vi "能谱拼接.vi"(1 "数组":string[](array[string])) -> (0 "拼接数组":i32[](array[numeric]))   [LabVIEW 2014]
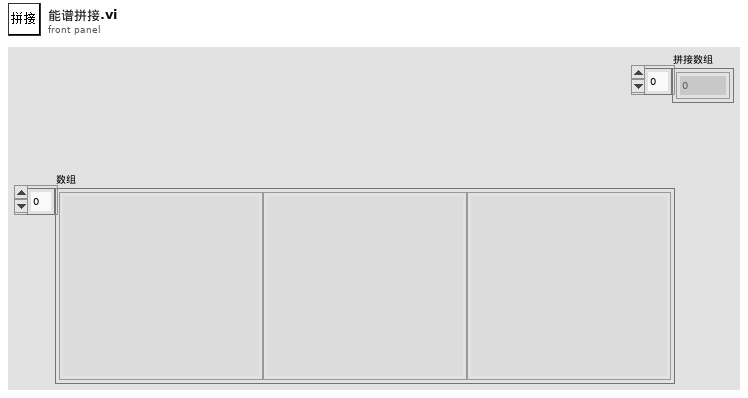
[diagram p1: front panel]
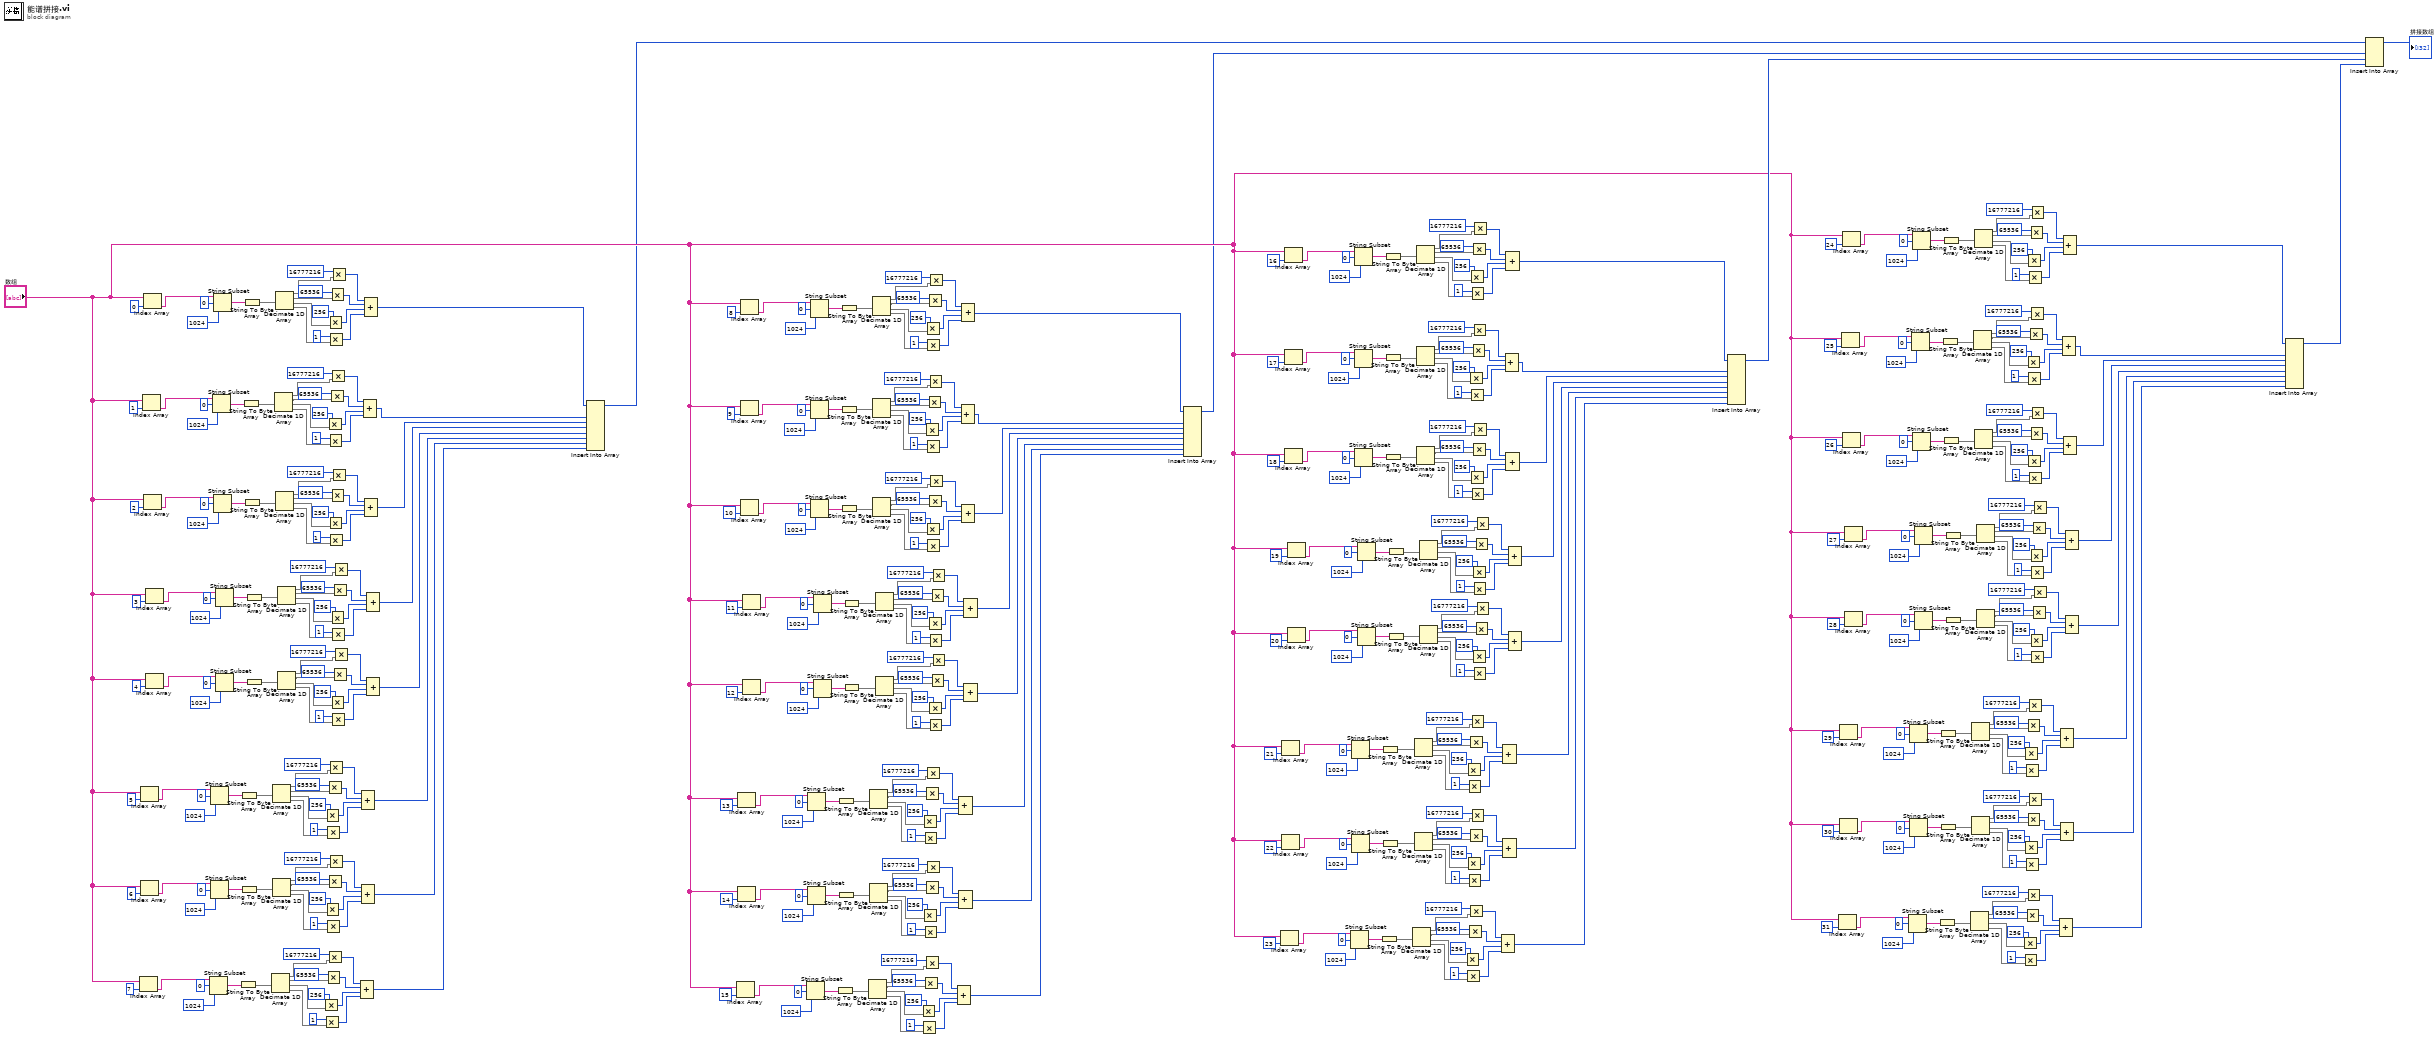
[diagram p0: block diagram]
diagram:
  n1 = Index Array(array="数组", index=7 ("索引")) -> (element=w465:string)
  n2 = Index Array(array="数组", index=5 ("索引")) -> (element=w503:string)
  n3 = Index Array(array="数组", index=6 ("索引")) -> (element=w484:string)
  n4 = Index Array(array="数组", index=1 ("索引")) -> (element=w579:string)
  n5 = Index Array(array="数组", index=0 ("索引")) -> (element=w598:string)
  n6 = Index Array(array="数组", index=2 ("索引")) -> (element=w560:string)
  n7 = Index Array(array="数组", index=3 ("索引")) -> (element=w541:string)
  n8 = Index Array(array="数组", index=4 ("索引")) -> (element=w522:string)
  n9 = String Subset(string=w465, offset (0)=0 ("偏移量(0)"), length (rest)=1024 ("长度（剩余）")) -> (substring=w479:string)
  n10 = String Subset(string=w503, offset (0)=0 ("偏移量(0)"), length (rest)=1024 ("长度（剩余）")) -> (substring=w517:string)
  n11 = String Subset(string=w484, offset (0)=0 ("偏移量(0)"), length (rest)=1024 ("长度（剩余）")) -> (substring=w498:string)
  n12 = String Subset(string=w579, offset (0)=0 ("偏移量(0)"), length (rest)=1024 ("长度（剩余）")) -> (substring=w593:string)
  n13 = String Subset(string=w598, offset (0)=0 ("偏移量(0)"), length (rest)=1024 ("长度（剩余）")) -> (substring=w612:string)
  n14 = String Subset(string=w560, offset (0)=0 ("偏移量(0)"), length (rest)=1024 ("长度（剩余）")) -> (substring=w574:string)
  n15 = String Subset(string=w541, offset (0)=0 ("偏移量(0)"), length (rest)=1024 ("长度（剩余）")) -> (substring=w555:string)
  n16 = String Subset(string=w522, offset (0)=0 ("偏移量(0)"), length (rest)=1024 ("长度（剩余）")) -> (substring=w536:string)
  n17 = String To Byte Array(string=w479) -> (unsigned byte array=w466:u8[])
  n18 = String To Byte Array(string=w517) -> (unsigned byte array=w504:u8[])
  n19 = String To Byte Array(string=w498) -> (unsigned byte array=w485:u8[])
  n20 = String To Byte Array(string=w593) -> (unsigned byte array=w580:u8[])
  n21 = String To Byte Array(string=w612) -> (unsigned byte array=w599:u8[])
  n22 = String To Byte Array(string=w574) -> (unsigned byte array=w561:u8[])
  n23 = String To Byte Array(string=w555) -> (unsigned byte array=w542:u8[])
  n24 = String To Byte Array(string=w536) -> (unsigned byte array=w523:u8[])
  n25 = Decimate 1D Array(w466) -> (w467:u8[], w468:u8[], w478:u8[], w477:u8[])
  n26 = Decimate 1D Array(w504) -> (w505:u8[], w506:u8[], w516:u8[], w515:u8[])
  n27 = Decimate 1D Array(w485) -> (w486:u8[], w487:u8[], w497:u8[], w496:u8[])
  n28 = Decimate 1D Array(w580) -> (w581:u8[], w582:u8[], w592:u8[], w591:u8[])
  n29 = Decimate 1D Array(w599) -> (w600:u8[], w601:u8[], w611:u8[], w610:u8[])
  n30 = Decimate 1D Array(w561) -> (w562:u8[], w563:u8[], w573:u8[], w572:u8[])
  n31 = Decimate 1D Array(w542) -> (w543:u8[], w544:u8[], w554:u8[], w553:u8[])
  n32 = Decimate 1D Array(w523) -> (w524:u8[], w525:u8[], w535:u8[], w534:u8[])
  n33 = Multiply(x=256, y=w478) -> (x*y=w473:i32[])
  n34 = Multiply(x=1, y=w477) -> (x*y=w474:i32[])
  n35 = Multiply(x=256, y=w516) -> (x*y=w511:i32[])
  n36 = Multiply(x=256, y=w497) -> (x*y=w492:i32[])
  n37 = Multiply(x=1, y=w515) -> (x*y=w512:i32[])
  n38 = Multiply(x=1, y=w496) -> (x*y=w493:i32[])
  n39 = Multiply(x=65536, y=w468) -> (x*y=w470:i32[])
  n40 = Multiply(x=256, y=w592) -> (x*y=w587:i32[])
  n41 = Multiply(x=65536, y=w506) -> (x*y=w508:i32[])
  n42 = Multiply(x=65536, y=w487) -> (x*y=w489:i32[])
  n43 = Multiply(x=16777216, y=w467) -> (x*y=w469:i32[])
  n44 = Multiply(x=256, y=w611) -> (x*y=w606:i32[])
  n45 = Multiply(x=1, y=w591) -> (x*y=w588:i32[])
  n46 = Multiply(x=256, y=w573) -> (x*y=w568:i32[])
  n47 = Multiply(x=1, y=w610) -> (x*y=w607:i32[])
  n48 = Multiply(x=1, y=w572) -> (x*y=w569:i32[])
  n49 = Multiply(x=16777216, y=w505) -> (x*y=w507:i32[])
  n50 = Multiply(x=16777216, y=w486) -> (x*y=w488:i32[])
  n51 = Multiply(x=65536, y=w582) -> (x*y=w584:i32[])
  n52 = Multiply(x=65536, y=w601) -> (x*y=w603:i32[])
  n53 = Multiply(x=65536, y=w563) -> (x*y=w565:i32[])
  n54 = Multiply(x=256, y=w554) -> (x*y=w549:i32[])
  n55 = Multiply(x=256, y=w535) -> (x*y=w530:i32[])
  n56 = Multiply(x=16777216, y=w581) -> (x*y=w583:i32[])
  n57 = Multiply(x=1, y=w553) -> (x*y=w550:i32[])
  n58 = Multiply(x=1, y=w534) -> (x*y=w531:i32[])
  n59 = Multiply(x=16777216, y=w600) -> (x*y=w602:i32[])
  n60 = Multiply(x=16777216, y=w562) -> (x*y=w564:i32[])
  n61 = Multiply(x=65536, y=w544) -> (x*y=w546:i32[])
  n62 = Multiply(x=65536, y=w525) -> (x*y=w527:i32[])
  n63 = Multiply(x=16777216, y=w543) -> (x*y=w545:i32[])
  n64 = Multiply(x=16777216, y=w524) -> (x*y=w526:i32[])
  n65 = Compound Arithmetic op=ADD(w469, w470, w473, w474) -> (w463:i32[])
  n66 = Compound Arithmetic op=ADD(w507, w508, w511, w512) -> (w501:i32[])
  n67 = Compound Arithmetic op=ADD(w488, w489, w492, w493) -> (w482:i32[])
  n68 = Compound Arithmetic op=ADD(w583, w584, w587, w588) -> (w577:i32[])
  n69 = Compound Arithmetic op=ADD(w602, w603, w606, w607) -> (w596:i32[])
  n70 = Compound Arithmetic op=ADD(w564, w565, w568, w569) -> (w558:i32[])
  n71 = Compound Arithmetic op=ADD(w545, w546, w549, w550) -> (w539:i32[])
  n72 = Compound Arithmetic op=ADD(w526, w527, w530, w531) -> (w520:i32[])
  n73 = Insert Into Array(array=w596, new element #1=w577, new element #2=w558, new element #3=w539, new element #4=w520, new element #5=w501, new element #6=w482, new element #7=w463) -> (w5:i32[])  [unwired: 1 in]
  n74 = Index Array(array="数组", index=15 ("索引")) -> (element=w314:string)
  n75 = Index Array(array="数组", index=13 ("索引")) -> (element=w352:string)
  n76 = Index Array(array="数组", index=14 ("索引")) -> (element=w333:string)
  n77 = Index Array(array="数组", index=9 ("索引")) -> (element=w428:string)
  n78 = Index Array(array="数组", index=8 ("索引")) -> (element=w447:string)
  n79 = Index Array(array="数组", index=10 ("索引")) -> (element=w409:string)
  n80 = Index Array(array="数组", index=11 ("索引")) -> (element=w390:string)
  n81 = Index Array(array="数组", index=12 ("索引")) -> (element=w371:string)
  n82 = String Subset(string=w314, offset (0)=0 ("偏移量(0)"), length (rest)=1024 ("长度（剩余）")) -> (substring=w328:string)
  n83 = String Subset(string=w352, offset (0)=0 ("偏移量(0)"), length (rest)=1024 ("长度（剩余）")) -> (substring=w366:string)
  n84 = String Subset(string=w333, offset (0)=0 ("偏移量(0)"), length (rest)=1024 ("长度（剩余）")) -> (substring=w347:string)
  n85 = String Subset(string=w428, offset (0)=0 ("偏移量(0)"), length (rest)=1024 ("长度（剩余）")) -> (substring=w442:string)
  n86 = String Subset(string=w447, offset (0)=0 ("偏移量(0)"), length (rest)=1024 ("长度（剩余）")) -> (substring=w460:string)
  n87 = String Subset(string=w409, offset (0)=0 ("偏移量(0)"), length (rest)=1024 ("长度（剩余）")) -> (substring=w423:string)
  n88 = String Subset(string=w390, offset (0)=0 ("偏移量(0)"), length (rest)=1024 ("长度（剩余）")) -> (substring=w404:string)
  n89 = String Subset(string=w371, offset (0)=0 ("偏移量(0)"), length (rest)=1024 ("长度（剩余）")) -> (substring=w385:string)
  n90 = String To Byte Array(string=w328) -> (unsigned byte array=w315:u8[])
  n91 = String To Byte Array(string=w366) -> (unsigned byte array=w353:u8[])
  n92 = String To Byte Array(string=w347) -> (unsigned byte array=w334:u8[])
  n93 = String To Byte Array(string=w442) -> (unsigned byte array=w429:u8[])
  n94 = String To Byte Array(string=w460) -> (unsigned byte array=w448:u8[])
  n95 = String To Byte Array(string=w423) -> (unsigned byte array=w410:u8[])
  n96 = String To Byte Array(string=w404) -> (unsigned byte array=w391:u8[])
  n97 = String To Byte Array(string=w385) -> (unsigned byte array=w372:u8[])
  n98 = Decimate 1D Array(w315) -> (w316:u8[], w317:u8[], w327:u8[], w326:u8[])
  n99 = Decimate 1D Array(w353) -> (w354:u8[], w355:u8[], w365:u8[], w364:u8[])
  n100 = Decimate 1D Array(w334) -> (w335:u8[], w336:u8[], w346:u8[], w345:u8[])
  n101 = Decimate 1D Array(w429) -> (w430:u8[], w431:u8[], w441:u8[], w440:u8[])
  n102 = Decimate 1D Array(w448) -> (w449:u8[], w450:u8[], w459:u8[], w458:u8[])
  n103 = Decimate 1D Array(w410) -> (w411:u8[], w412:u8[], w422:u8[], w421:u8[])
  n104 = Decimate 1D Array(w391) -> (w392:u8[], w393:u8[], w403:u8[], w402:u8[])
  n105 = Decimate 1D Array(w372) -> (w373:u8[], w374:u8[], w384:u8[], w383:u8[])
  n106 = Multiply(x=256, y=w327) -> (x*y=w322:i32[])
  n107 = Multiply(x=1, y=w326) -> (x*y=w323:i32[])
  n108 = Multiply(x=256, y=w365) -> (x*y=w360:i32[])
  n109 = Multiply(x=256, y=w346) -> (x*y=w341:i32[])
  n110 = Multiply(x=1, y=w364) -> (x*y=w361:i32[])
  n111 = Multiply(x=1, y=w345) -> (x*y=w342:i32[])
  n112 = Multiply(x=65536, y=w317) -> (x*y=w319:i32[])
  n113 = Multiply(x=256, y=w441) -> (x*y=w436:i32[])
  n114 = Multiply(x=65536, y=w355) -> (x*y=w357:i32[])
  n115 = Multiply(x=65536, y=w336) -> (x*y=w338:i32[])
  n116 = Multiply(x=16777216, y=w316) -> (x*y=w318:i32[])
  n117 = Multiply(x=256, y=w459) -> (x*y=w454:i32[])
  n118 = Multiply(x=1, y=w440) -> (x*y=w437:i32[])
  n119 = Multiply(x=256, y=w422) -> (x*y=w417:i32[])
  n120 = Multiply(x=1, y=w458) -> (x*y=w455:i32[])
  n121 = Multiply(x=1, y=w421) -> (x*y=w418:i32[])
  n122 = Multiply(x=16777216, y=w354) -> (x*y=w356:i32[])
  n123 = Multiply(x=16777216, y=w335) -> (x*y=w337:i32[])
  n124 = Multiply(x=65536, y=w431) -> (x*y=w433:i32[])
  n125 = Multiply(x=65536, y=w450) -> (x*y=w452:i32[])
  n126 = Multiply(x=65536, y=w412) -> (x*y=w414:i32[])
  n127 = Multiply(x=256, y=w403) -> (x*y=w398:i32[])
  n128 = Multiply(x=256, y=w384) -> (x*y=w379:i32[])
  n129 = Multiply(x=16777216, y=w430) -> (x*y=w432:i32[])
  n130 = Multiply(x=1, y=w402) -> (x*y=w399:i32[])
  n131 = Multiply(x=1, y=w383) -> (x*y=w380:i32[])
  n132 = Multiply(x=16777216, y=w449) -> (x*y=w451:i32[])
  n133 = Multiply(x=16777216, y=w411) -> (x*y=w413:i32[])
  n134 = Multiply(x=65536, y=w393) -> (x*y=w395:i32[])
  n135 = Multiply(x=65536, y=w374) -> (x*y=w376:i32[])
  n136 = Multiply(x=16777216, y=w392) -> (x*y=w394:i32[])
  n137 = Multiply(x=16777216, y=w373) -> (x*y=w375:i32[])
  n138 = Compound Arithmetic op=ADD(w318, w319, w322, w323) -> (w312:i32[])
  n139 = Compound Arithmetic op=ADD(w356, w357, w360, w361) -> (w350:i32[])
  n140 = Compound Arithmetic op=ADD(w337, w338, w341, w342) -> (w331:i32[])
  n141 = Compound Arithmetic op=ADD(w432, w433, w436, w437) -> (w426:i32[])
  n142 = Compound Arithmetic op=ADD(w451, w452, w454, w455) -> (w445:i32[])
  n143 = Compound Arithmetic op=ADD(w413, w414, w417, w418) -> (w407:i32[])
  n144 = Compound Arithmetic op=ADD(w394, w395, w398, w399) -> (w388:i32[])
  n145 = Compound Arithmetic op=ADD(w375, w376, w379, w380) -> (w369:i32[])
  n146 = Insert Into Array(array=w445, new element #1=w426, new element #2=w407, new element #3=w388, new element #4=w369, new element #5=w350, new element #6=w331, new element #7=w312) -> (w6:i32[])  [unwired: 1 in]
  n147 = Index Array(array="数组", index=23 ("索引")) -> (element=w163:string)
  n148 = Index Array(array="数组", index=21 ("索引")) -> (element=w201:string)
  n149 = Index Array(array="数组", index=22 ("索引")) -> (element=w182:string)
  n150 = Index Array(array="数组", index=17 ("索引")) -> (element=w277:string)
  n151 = Index Array(array="数组", index=16 ("索引")) -> (element=w296:string)
  n152 = Index Array(array="数组", index=18 ("索引")) -> (element=w258:string)
  n153 = Index Array(array="数组", index=19 ("索引")) -> (element=w239:string)
  n154 = Index Array(array="数组", index=20 ("索引")) -> (element=w220:string)
  n155 = String Subset(string=w163, offset (0)=0 ("偏移量(0)"), length (rest)=1024 ("长度（剩余）")) -> (substring=w177:string)
  n156 = String Subset(string=w201, offset (0)=0 ("偏移量(0)"), length (rest)=1024 ("长度（剩余）")) -> (substring=w215:string)
  n157 = String Subset(string=w182, offset (0)=0 ("偏移量(0)"), length (rest)=1024 ("长度（剩余）")) -> (substring=w196:string)
  n158 = String Subset(string=w277, offset (0)=0 ("偏移量(0)"), length (rest)=1024 ("长度（剩余）")) -> (substring=w291:string)
  n159 = String Subset(string=w296, offset (0)=0 ("偏移量(0)"), length (rest)=1024 ("长度（剩余）")) -> (substring=w309:string)
  n160 = String Subset(string=w258, offset (0)=0 ("偏移量(0)"), length (rest)=1024 ("长度（剩余）")) -> (substring=w272:string)
  n161 = String Subset(string=w239, offset (0)=0 ("偏移量(0)"), length (rest)=1024 ("长度（剩余）")) -> (substring=w253:string)
  n162 = String Subset(string=w220, offset (0)=0 ("偏移量(0)"), length (rest)=1024 ("长度（剩余）")) -> (substring=w234:string)
  n163 = String To Byte Array(string=w177) -> (unsigned byte array=w164:u8[])
  n164 = String To Byte Array(string=w215) -> (unsigned byte array=w202:u8[])
  n165 = String To Byte Array(string=w196) -> (unsigned byte array=w183:u8[])
  n166 = String To Byte Array(string=w291) -> (unsigned byte array=w278:u8[])
  n167 = String To Byte Array(string=w309) -> (unsigned byte array=w297:u8[])
  n168 = String To Byte Array(string=w272) -> (unsigned byte array=w259:u8[])
  n169 = String To Byte Array(string=w253) -> (unsigned byte array=w240:u8[])
  n170 = String To Byte Array(string=w234) -> (unsigned byte array=w221:u8[])
  n171 = Decimate 1D Array(w164) -> (w165:u8[], w166:u8[], w176:u8[], w175:u8[])
  n172 = Decimate 1D Array(w202) -> (w203:u8[], w204:u8[], w214:u8[], w213:u8[])
  n173 = Decimate 1D Array(w183) -> (w184:u8[], w185:u8[], w195:u8[], w194:u8[])
  n174 = Decimate 1D Array(w278) -> (w279:u8[], w280:u8[], w290:u8[], w289:u8[])
  n175 = Decimate 1D Array(w297) -> (w298:u8[], w299:u8[], w308:u8[], w307:u8[])
  n176 = Decimate 1D Array(w259) -> (w260:u8[], w261:u8[], w271:u8[], w270:u8[])
  n177 = Decimate 1D Array(w240) -> (w241:u8[], w242:u8[], w252:u8[], w251:u8[])
  n178 = Decimate 1D Array(w221) -> (w222:u8[], w223:u8[], w233:u8[], w232:u8[])
  n179 = Multiply(x=256, y=w176) -> (x*y=w171:i32[])
  n180 = Multiply(x=1, y=w175) -> (x*y=w172:i32[])
  n181 = Multiply(x=256, y=w214) -> (x*y=w209:i32[])
  n182 = Multiply(x=256, y=w195) -> (x*y=w190:i32[])
  n183 = Multiply(x=1, y=w213) -> (x*y=w210:i32[])
  n184 = Multiply(x=1, y=w194) -> (x*y=w191:i32[])
  n185 = Multiply(x=65536, y=w166) -> (x*y=w168:i32[])
  n186 = Multiply(x=256, y=w290) -> (x*y=w285:i32[])
  n187 = Multiply(x=65536, y=w204) -> (x*y=w206:i32[])
  n188 = Multiply(x=65536, y=w185) -> (x*y=w187:i32[])
  n189 = Multiply(x=16777216, y=w165) -> (x*y=w167:i32[])
  n190 = Multiply(x=256, y=w308) -> (x*y=w303:i32[])
  n191 = Multiply(x=1, y=w289) -> (x*y=w286:i32[])
  n192 = Multiply(x=256, y=w271) -> (x*y=w266:i32[])
  n193 = Multiply(x=1, y=w307) -> (x*y=w304:i32[])
  n194 = Multiply(x=1, y=w270) -> (x*y=w267:i32[])
  n195 = Multiply(x=16777216, y=w203) -> (x*y=w205:i32[])
  n196 = Multiply(x=16777216, y=w184) -> (x*y=w186:i32[])
  n197 = Multiply(x=65536, y=w280) -> (x*y=w282:i32[])
  n198 = Multiply(x=65536, y=w299) -> (x*y=w301:i32[])
  n199 = Multiply(x=65536, y=w261) -> (x*y=w263:i32[])
  n200 = Multiply(x=256, y=w252) -> (x*y=w247:i32[])
  n201 = Multiply(x=256, y=w233) -> (x*y=w228:i32[])
  n202 = Multiply(x=16777216, y=w279) -> (x*y=w281:i32[])
  n203 = Multiply(x=1, y=w251) -> (x*y=w248:i32[])
  n204 = Multiply(x=1, y=w232) -> (x*y=w229:i32[])
  n205 = Multiply(x=16777216, y=w298) -> (x*y=w300:i32[])
  n206 = Multiply(x=16777216, y=w260) -> (x*y=w262:i32[])
  n207 = Multiply(x=65536, y=w242) -> (x*y=w244:i32[])
  n208 = Multiply(x=65536, y=w223) -> (x*y=w225:i32[])
  n209 = Multiply(x=16777216, y=w241) -> (x*y=w243:i32[])
  n210 = Multiply(x=16777216, y=w222) -> (x*y=w224:i32[])
  n211 = Compound Arithmetic op=ADD(w167, w168, w171, w172) -> (w161:i32[])
  n212 = Compound Arithmetic op=ADD(w205, w206, w209, w210) -> (w199:i32[])
  n213 = Compound Arithmetic op=ADD(w186, w187, w190, w191) -> (w180:i32[])
  n214 = Compound Arithmetic op=ADD(w281, w282, w285, w286) -> (w275:i32[])
  n215 = Compound Arithmetic op=ADD(w300, w301, w303, w304) -> (w294:i32[])
  n216 = Compound Arithmetic op=ADD(w262, w263, w266, w267) -> (w256:i32[])
  n217 = Compound Arithmetic op=ADD(w243, w244, w247, w248) -> (w237:i32[])
  n218 = Compound Arithmetic op=ADD(w224, w225, w228, w229) -> (w218:i32[])
  n219 = Insert Into Array(array=w294, new element #1=w275, new element #2=w256, new element #3=w237, new element #4=w218, new element #5=w199, new element #6=w180, new element #7=w161) -> (w8:i32[])  [unwired: 1 in]
  n220 = Index Array(array="数组", index=31 ("索引")) -> (element=w12:string)
  n221 = Index Array(array="数组", index=29 ("索引")) -> (element=w50:string)
  n222 = Index Array(array="数组", index=30 ("索引")) -> (element=w31:string)
  n223 = Index Array(array="数组", index=25 ("索引")) -> (element=w126:string)
  n224 = Index Array(array="数组", index=24 ("索引")) -> (element=w145:string)
  n225 = Index Array(array="数组", index=26 ("索引")) -> (element=w107:string)
  n226 = Index Array(array="数组", index=27 ("索引")) -> (element=w88:string)
  n227 = Index Array(array="数组", index=28 ("索引")) -> (element=w69:string)
  n228 = String Subset(string=w12, offset (0)=0 ("偏移量(0)"), length (rest)=1024 ("长度（剩余）")) -> (substring=w26:string)
  n229 = String Subset(string=w50, offset (0)=0 ("偏移量(0)"), length (rest)=1024 ("长度（剩余）")) -> (substring=w64:string)
  n230 = String Subset(string=w31, offset (0)=0 ("偏移量(0)"), length (rest)=1024 ("长度（剩余）")) -> (substring=w45:string)
  n231 = String Subset(string=w126, offset (0)=0 ("偏移量(0)"), length (rest)=1024 ("长度（剩余）")) -> (substring=w140:string)
  n232 = String Subset(string=w145, offset (0)=0 ("偏移量(0)"), length (rest)=1024 ("长度（剩余）")) -> (substring=w158:string)
  n233 = String Subset(string=w107, offset (0)=0 ("偏移量(0)"), length (rest)=1024 ("长度（剩余）")) -> (substring=w121:string)
  n234 = String Subset(string=w88, offset (0)=0 ("偏移量(0)"), length (rest)=1024 ("长度（剩余）")) -> (substring=w102:string)
  n235 = String Subset(string=w69, offset (0)=0 ("偏移量(0)"), length (rest)=1024 ("长度（剩余）")) -> (substring=w83:string)
  n236 = String To Byte Array(string=w26) -> (unsigned byte array=w13:u8[])
  n237 = String To Byte Array(string=w64) -> (unsigned byte array=w51:u8[])
  n238 = String To Byte Array(string=w45) -> (unsigned byte array=w32:u8[])
  n239 = String To Byte Array(string=w140) -> (unsigned byte array=w127:u8[])
  n240 = String To Byte Array(string=w158) -> (unsigned byte array=w146:u8[])
  n241 = String To Byte Array(string=w121) -> (unsigned byte array=w108:u8[])
  n242 = String To Byte Array(string=w102) -> (unsigned byte array=w89:u8[])
  n243 = String To Byte Array(string=w83) -> (unsigned byte array=w70:u8[])
  n244 = Decimate 1D Array(w13) -> (w14:u8[], w15:u8[], w25:u8[], w24:u8[])
  n245 = Decimate 1D Array(w51) -> (w52:u8[], w53:u8[], w63:u8[], w62:u8[])
  n246 = Decimate 1D Array(w32) -> (w33:u8[], w34:u8[], w44:u8[], w43:u8[])
  n247 = Decimate 1D Array(w127) -> (w128:u8[], w129:u8[], w139:u8[], w138:u8[])
  n248 = Decimate 1D Array(w146) -> (w147:u8[], w148:u8[], w157:u8[], w156:u8[])
  n249 = Decimate 1D Array(w108) -> (w109:u8[], w110:u8[], w120:u8[], w119:u8[])
  n250 = Decimate 1D Array(w89) -> (w90:u8[], w91:u8[], w101:u8[], w100:u8[])
  n251 = Decimate 1D Array(w70) -> (w71:u8[], w72:u8[], w82:u8[], w81:u8[])
  n252 = Multiply(x=256, y=w25) -> (x*y=w20:i32[])
  n253 = Multiply(x=1, y=w24) -> (x*y=w21:i32[])
  n254 = Multiply(x=256, y=w63) -> (x*y=w58:i32[])
  n255 = Multiply(x=256, y=w44) -> (x*y=w39:i32[])
  n256 = Multiply(x=1, y=w62) -> (x*y=w59:i32[])
  n257 = Multiply(x=1, y=w43) -> (x*y=w40:i32[])
  n258 = Multiply(x=65536, y=w15) -> (x*y=w17:i32[])
  n259 = Multiply(x=256, y=w139) -> (x*y=w134:i32[])
  n260 = Multiply(x=65536, y=w53) -> (x*y=w55:i32[])
  n261 = Multiply(x=65536, y=w34) -> (x*y=w36:i32[])
  n262 = Multiply(x=16777216, y=w14) -> (x*y=w16:i32[])
  n263 = Multiply(x=256, y=w157) -> (x*y=w152:i32[])
  n264 = Multiply(x=1, y=w138) -> (x*y=w135:i32[])
  n265 = Multiply(x=256, y=w120) -> (x*y=w115:i32[])
  n266 = Multiply(x=1, y=w156) -> (x*y=w153:i32[])
  n267 = Multiply(x=1, y=w119) -> (x*y=w116:i32[])
  n268 = Multiply(x=16777216, y=w52) -> (x*y=w54:i32[])
  n269 = Multiply(x=16777216, y=w33) -> (x*y=w35:i32[])
  n270 = Multiply(x=65536, y=w129) -> (x*y=w131:i32[])
  n271 = Multiply(x=65536, y=w148) -> (x*y=w150:i32[])
  n272 = Multiply(x=65536, y=w110) -> (x*y=w112:i32[])
  n273 = Multiply(x=256, y=w101) -> (x*y=w96:i32[])
  n274 = Multiply(x=256, y=w82) -> (x*y=w77:i32[])
  n275 = Multiply(x=16777216, y=w128) -> (x*y=w130:i32[])
  n276 = Multiply(x=1, y=w100) -> (x*y=w97:i32[])
  n277 = Multiply(x=1, y=w81) -> (x*y=w78:i32[])
  n278 = Multiply(x=16777216, y=w147) -> (x*y=w149:i32[])
  n279 = Multiply(x=16777216, y=w109) -> (x*y=w111:i32[])
  n280 = Multiply(x=65536, y=w91) -> (x*y=w93:i32[])
  n281 = Multiply(x=65536, y=w72) -> (x*y=w74:i32[])
  n282 = Multiply(x=16777216, y=w90) -> (x*y=w92:i32[])
  n283 = Multiply(x=16777216, y=w71) -> (x*y=w73:i32[])
  n284 = Compound Arithmetic op=ADD(w16, w17, w20, w21) -> (w10:i32[])
  n285 = Compound Arithmetic op=ADD(w54, w55, w58, w59) -> (w48:i32[])
  n286 = Compound Arithmetic op=ADD(w35, w36, w39, w40) -> (w29:i32[])
  n287 = Compound Arithmetic op=ADD(w130, w131, w134, w135) -> (w124:i32[])
  n288 = Compound Arithmetic op=ADD(w149, w150, w152, w153) -> (w143:i32[])
  n289 = Compound Arithmetic op=ADD(w111, w112, w115, w116) -> (w105:i32[])
  n290 = Compound Arithmetic op=ADD(w92, w93, w96, w97) -> (w86:i32[])
  n291 = Compound Arithmetic op=ADD(w73, w74, w77, w78) -> (w67:i32[])
  n292 = Insert Into Array(array=w143, new element #1=w124, new element #2=w105, new element #3=w86, new element #4=w67, new element #5=w48, new element #6=w29, new element #7=w10) -> (w9:i32[])  [unwired: 1 in]
  n293 = Insert Into Array(array=w5, new element #1=w6, new element #2=w8, new element #3=w9) -> (→"拼接数组":i32[])  [unwired: 1 in]
